vi "Test Find Homography.vi"(11 "Test Case In":refnum<class "03_AR.lvclass">) -> (0 "error out":errorcluster, 3 "Test Case Out":refnum<class "03_AR.lvclass">)   [LabVIEW 2020, in "test.lvlib" / "03_AR.lvclass"]
uses:
  03_AR.lvclass
  C:/Program Files (x86)/National Instruments/LabVIEW 2026/vi.lib/Astemes/LUnit/Test Case.lvclass
  common/Image Point (Float).ctl
  <vilib>/Analysis/Matrix/Datatypes/RealMatrix.ctl
  ar/USAC Params/USAC Params.lvclass/USAC Params.ctl
  <vilib>/Astemes/LUnit/Test Case.lvclass/Test Case.ctl
  4993e8ee-a06a-463a-9684-69129f64d5ce.vi
  a9e8ae8b-571d-475d-bf6f-113481f926df.vi
  ar/USAC Params/Get Params.vi
  <vilib>/Astemes/LUnit/Core/LUnit Test Case/Private/Append Pass Result.vi
  <vilib>/Astemes/LUnit/Core/LUnit Test Case/Private/Append Fail Result.vi
  4993e8ee-a06a-463a-9684-69129f64d5ce.vi/9c5d11cd-9439-4240-a1ee-d9baace9c924.vi
  a9e8ae8b-571d-475d-bf6f-113481f926df.vi/9c5d11cd-9439-4240-a1ee-d9baace9c924.vi
  <vilib>/Astemes/LUnit/Core/LUnit Test Case/Private/Run In UI.vi
  <vilib>/Utility/error.llb/Clear Errors.vi
  <vilib>/Analysis/Matrix/Numeric/Conversions/Array To Matrix.vi
  <vilib>/Analysis/Matrix/Numeric/Conversions/Array To Matrix - RA2.vi
  <vilib>/Utility/error.llb/Error Cluster From Error Code.vi
  <vilib>/Analysis/Matrix/Comparison/Equal/Equal.vi
  <vilib>/Analysis/Matrix/Comparison/Equal/Equal - RM,RM.vi
  ar/USAC Params/USAC Params.lvclass
  ar/ar.lvlib
  common/common.lvlib
  <vilib>/Analysis/Matrix/NI_Matrix.lvlib
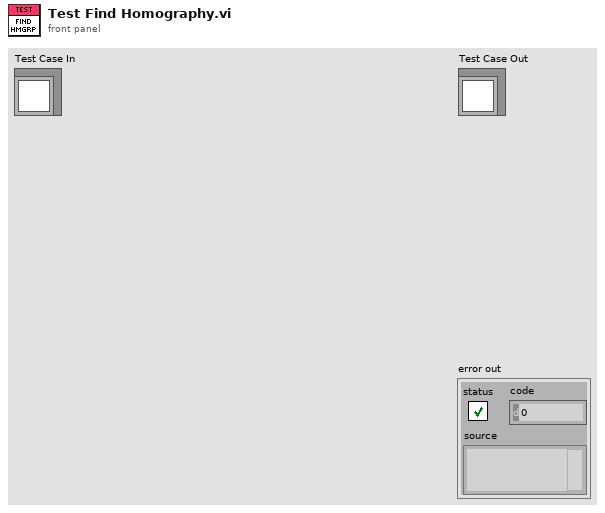
[diagram p1: front panel]
types:
  T1 = typedef "NI_Matrix.lvlib/RealMatrix.ctl" = dbl[][]
  T2 = typedef "common.lvlib/Image Point (Float).ctl" = cluster{"x":dbl, "y":dbl}
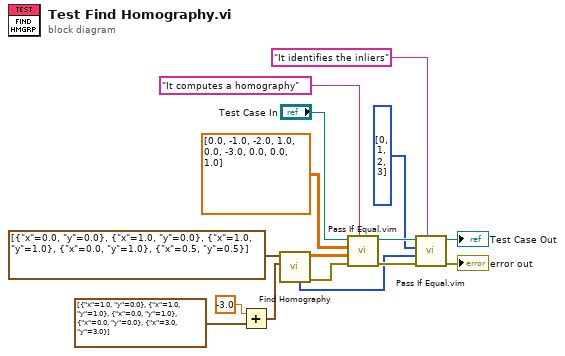
[diagram p0: block diagram]
diagram:
  n1 = Add(x=-3.0, y=T2[] [{"x"=1.0, "y"=0.0}, {"x"=1.0, "y"=1.0}, {"x"=0.0, "y"=1.0}, {"x"=0.0, "y"=0.0}, {"x"=3.0, "y"=3.0}] ("Target Points")) -> (x+y=w13:T2[])
  n2 = call "Find Homography.vi"("Target Points"=w13, "Source Points"=T2[] [{"x"=0.0, "y"=0.0}, {"x"=1.0, "y"=0.0}, {"x"=1.0, "y"=1.0}, {"x"=0.0, "y"=1.0}, {"x"=0.5, "y"=0.5}]) -> ("error out"=w11:errorcluster, "Homography Matrix"=w9:T1, "Inliers"=w3:i32[])  [unwired: 7 in]
  n3 = call "Pass If Equal.vim"("Description"="It computes a homography", "error in (no error)"=w11, "Actual"=w9, "Expected"=T1 [[0.0, -1.0, -2.0], [1.0, 0.0, -3.0], [0.0, 0.0, 1.0]] ("Homography Matrix 2"), "LUnit Test Case In"="Test Case In") -> ("error out"=w7:errorcluster, "LUnit Test Case Out"=w8:refnum<class "03_AR.lvclass">)  [unwired: 5 in]
  n4 = call "Pass If Equal.vim"("Description"="It identifies the inliers", "error in (no error)"=w7, "Actual"=w3, "Expected"=i32[] [0, 1, 2, 3] ("Inliers"), "LUnit Test Case In"=w8) -> ("error out"=→"error out":errorcluster, "LUnit Test Case Out"=→"Test Case Out":refnum<class "03_AR.lvclass">)  [unwired: 5 in]
